vi "Remove Element by Index.vi"(8 "error in (no error)":errorcluster, 10 "Index":i32, 11 "MusicElementLibrary":refnum<class "MusicElementLibrary.lvclass">) -> (0 "error out":errorcluster, 3 "MusicElementLibrary":refnum<class "MusicElementLibrary.lvclass">, 5 "Removed?":bool)   [LabVIEW 2015, in "MusicElementLibrary.lvclass"]
uses:
  MusicElementLibrary.lvclass
  MusicElementLibrary.lvclass/MusicElementLibrary.ctl
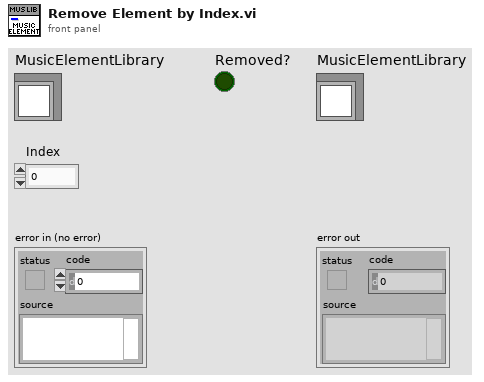
[diagram p1: front panel]
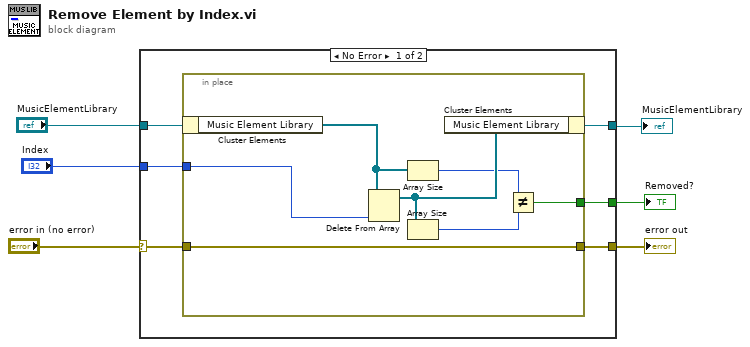
[diagram p0: block diagram]
diagram:
  n1 = case shown="No Error" "error in (no error)" {
    selector: "error in (no error)" -> [w12 w21]
    tunnel: [w8 w21] -> w5
    tunnel: [w10 w20] -> w2
    tunnel: "MusicElementLibrary" -> [w11 w20]
    tunnel: "Index" -> [w9 _]
    tunnel: [w7 _] -> w1
    frame No Error {
      n2 = in-place {
        in-place-border: w12 -> [w18]
        in-place-border: w9 -> [w19]
        in-place-border: [w18] -> w8
        in-place-border: [w13] -> w7
        n3 = in-place-cluster #1(w11) -> ("Music Element Library"=w16:refnum<class "MusicElement.lvclass">[])
        n4 = Delete From Array(array=w16, index=w19) -> (array with subset deleted=w17:refnum<class "MusicElement.lvclass">[])  [unwired: 1 in, 1 out]
        n5 = Array Size(array=w16) -> (size(s)=w15:i32)
        n6 = Array Size(array=w17) -> (size(s)=w14:i32)
        n7 = in-place-cluster #1("Music Element Library"=w17) -> (w10:refnum<class "MusicElementLibrary.lvclass">)
        n8 = Not Equal?(x=w15, y=w14) -> (x != y?=w13:bool)
      }
    }
    frame Error {
    }
  }
  "error out" <- w5
  "MusicElementLibrary" <- w2
  "Removed?" <- w1
